vi "BRig_RT__Case_Idle__calc_LaserPulse.vi"(4 "input_dataExp_L_Tshutter":i32, 6 "input_dataExp_L_Tpeak":i32, 8 "input_dataExp_L_T":i32, 9 "input_dataExp_L_freq":i32, 11 "input_dataExp":u16[](array[numeric])) -> (2 "output_cluster":cluster{u16[], u16[]})   [LabVIEW 2014]
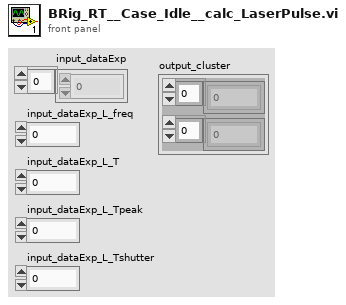
[diagram p1: front panel]
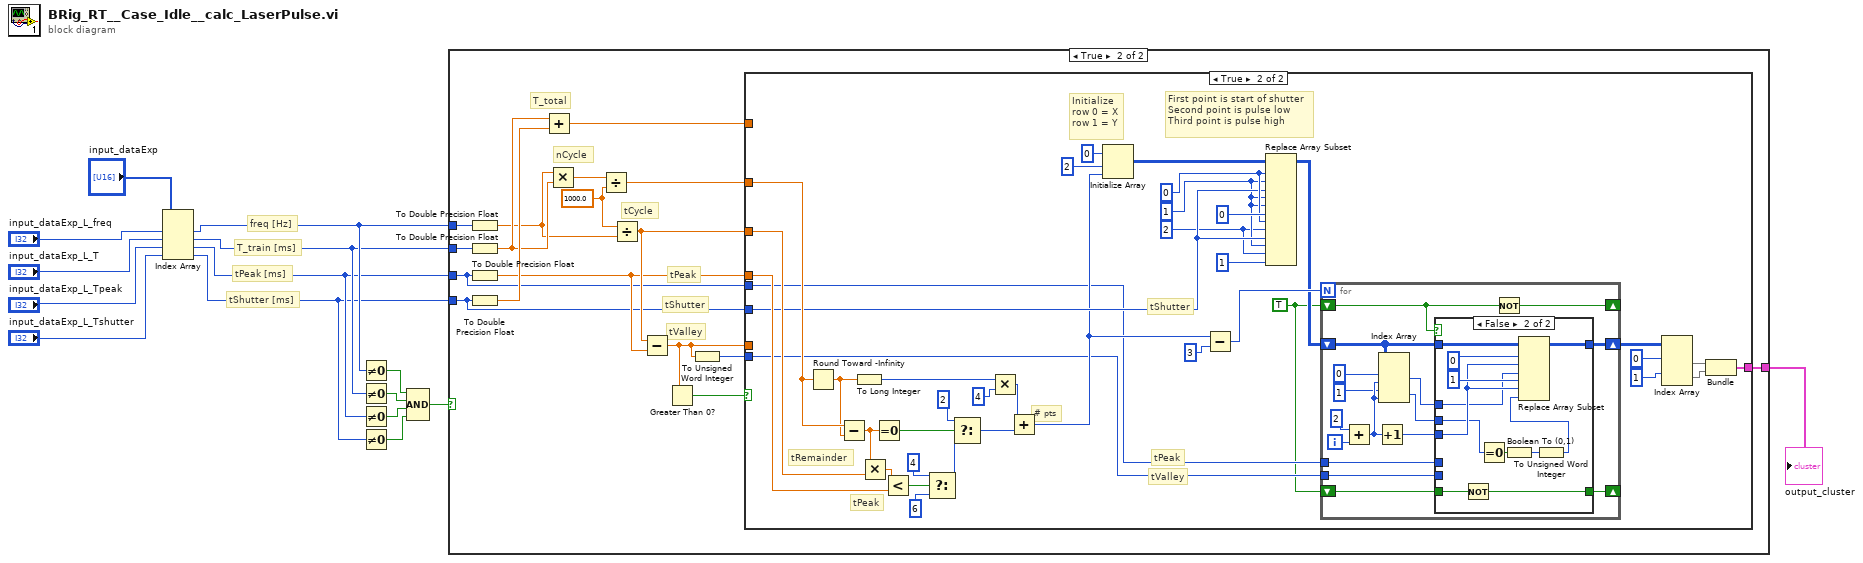
[diagram p0: block diagram]
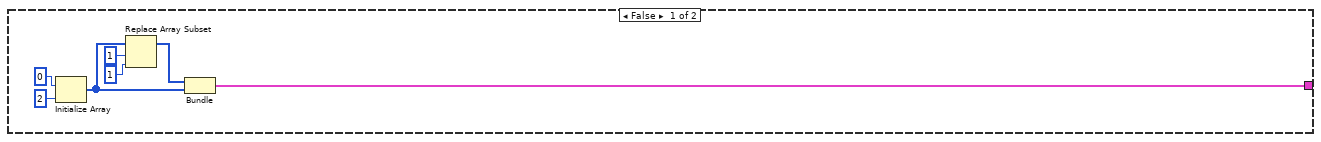
[diagram p2: hidden frame]
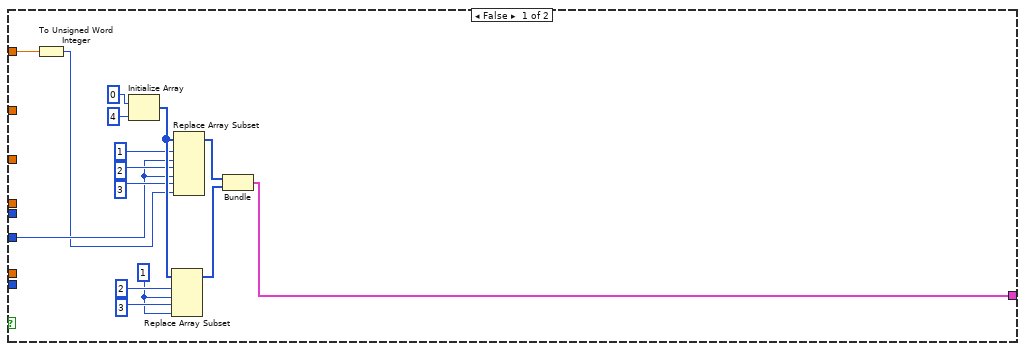
[diagram p3: hidden frame]
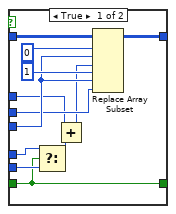
[diagram p4: hidden frame]
diagram:
  # "tShutter [ms]"
  # "tPeak [ms]"
  # "T_train [ms]"
  # "freq [Hz]"
  n1 = Index Array(array="input_dataExp", index #1="input_dataExp_L_freq", index #2="input_dataExp_L_T", index #3="input_dataExp_L_Tpeak", index #4="input_dataExp_L_Tshutter") -> (element #1=w8:u16, element #2=w7:u16, element #3=w6:u16, element #4=w5:u16)
  n2 = Not Equal To 0?(x=w8) -> (x != 0?=w14:bool)
  n3 = Not Equal To 0?(x=w7) -> (x != 0?=w13:bool)
  n4 = Not Equal To 0?(x=w6) -> (x != 0?=w12:bool)
  n5 = Not Equal To 0?(x=w5) -> (x != 0?=w11:bool)
  n6 = Compound Arithmetic op=AND(w14, w13, w12, w11) -> (w10:bool)
  n7 = case shown="True" w10 {
    tunnel: w8 -> [_ w34]
    tunnel: w7 -> [_ w33]
    tunnel: w6 -> [_ w26]
    tunnel: w5 -> [_ w27]
    tunnel: [w16 w23] -> w9
    frame False {
      n8 = Initialize Array(u16 0 ("element"), 2 ("dimension size")) -> (w20:u16[])
      n9 = Replace Array Subset(array=w20, new element=u16 1 ("new element/subarray"), index=1) -> (w17:u16[])
      n10 = Bundle(w17, w20) -> (w16:cluster{u16[], u16[]})  [unwired: 1 in]
    }
    frame True {
      w36 = 1000.0 ("y")
      # "tShutter"
      # "tPeak"
      # "tValley"
      # "tCycle"
      # "nCycle"
      # "T_total"
      n11 = To Double Precision Float(number=w34) -> (double precision float=w35:dbl)
      n12 = To Double Precision Float(number=w33) -> (double precision float=w38:dbl)
      n13 = To Double Precision Float(number=w26) -> (double precision float=w28:dbl)
      n14 = To Double Precision Float(number=w27) -> (double precision float=w39:dbl)
      n15 = Add(x=w38, y=w39) -> (x+y=w29:dbl)
      n16 = Multiply(x=w35, y=w38) -> (x*y=w37:dbl)
      n17 = Divide(x=w37, y=w36) -> (x/y=w30:dbl)
      n18 = Divide(x=w36, y=w35) -> (x/y=w31:dbl)
      n19 = Subtract(x=w31, y=w28) -> (x-y=w25:dbl)
      n20 = Greater Than 0?(x=w25) -> (x > 0?=w32:bool)
      n21 = To Unsigned Word Integer(number=w25) -> (unsigned 16bit integer=w24:u16)
      n22 = case shown="True" w32 {
        tunnel: w25 -> [_ _]
        tunnel: w31 -> [_ w89]
        tunnel: w30 -> [_ w79]
        tunnel: w29 -> [w43 _]
        tunnel: w28 -> [_ w87]
        tunnel: w27 -> [w44 w71]
        tunnel: w26 -> [_ w63]
        tunnel: w24 -> [_ w62]
        tunnel: [w40 w55] -> w23
        frame False {
          w50 = u16 1 ("new element/subarray")
          n23 = To Unsigned Word Integer(number=w43) -> (unsigned 16bit integer=w42:u16)
          n24 = Initialize Array(u16 0 ("element"), 4 ("dimension size")) -> (w48:u16[])
          n25 = Replace Array Subset(array=w48, new element #1=w50, index #1=2 ("index"), new element #2=w50, index #2=3 ("index")) -> (w49:u16[])
          n26 = Replace Array Subset(array=w48, new element #1=w44, index #1=1 ("new element/subarray"), new element #2=w44, index #2=2 ("index"), new element #3=w42, index #3=3 ("index")) -> (w41:u16[])
          n27 = Bundle(w41, w49) -> (w40:cluster{u16[], u16[]})  [unwired: 1 in]
        }
        frame True {
          w61 = TRUE
          w69 = 2 ("disabled index (col)")
          w70 = 1 ("dimension size")
          w72 = 0 ("dimension size")
          # "tValley"
          # "tPeak"
          # "tShutter"
          # "First point is start of shutter\nSecond point is pulse low\nThird point is pulse high"
          # "Initialize\nrow 0 = X\nrow 1 = Y"
          # "tPeak"
          # "tRemainder"
          # "# pts"
          n28 = Round Toward -Infinity(1:w79) -> (0:w78:dbl)
          n29 = Subtract(x=w79, y=w78) -> (x-y=w90:dbl)
          n30 = To Long Integer(number=w78) -> (32bit integer=w77:i32)
          n31 = Multiply(x=w90, y=w89) -> (x*y=w88:dbl)
          n32 = Equal To 0?(x=w90) -> (x = 0?=w92:bool)
          n33 = Less?(x=w88, y=w87) -> (x < y?=w86:bool)
          n34 = Select(t=4, s=w86, f=6) -> (s? t:f=w83:i32)
          n35 = Select(t=2, s=w92, f=w83) -> (s? t:f=w81:i32)
          n36 = Multiply(x=w77, y=4) -> (x*y=w80:i32)
          n37 = Add(x=w80, y=w81) -> (x+y=w67:i32)
          n38 = Initialize Array(u16 0 ("element"), 2 ("dimension size"), w67) -> (w74:u16[][])
          n39 = Subtract(x=w67, y=3) -> (x-y=w66:i32)
          n40 = Replace Array Subset(array=w74, new element #1=w71, index (row) #1=w72, index (col) #1=w70, new element #2=u16 0 ("new element/subarray"), index (row) #2=w70, index (col) #2=w70, new element #3=w71, index (row) #3=w72, index (col) #3=w69, new element #4=u16 1 ("new element/subarray"), index (row) #4=w70, index (col) #4=w69) -> (w64:u16[][])
          n41 = for {
            N: w66 -> [_]
            shift-right: [w93] -> w60
            shift-left: w64 -> [w101]
            tunnel: w63 -> [w97]
            tunnel: w62 -> [w96]
            shift-right: [w103] -> _
            shift-left: w61 -> [w102]
            shift-right: [w94] -> _
            shift-left: w61 -> [w95]
            i -> [w108]
            n42 = Add(x=2, y=w108) -> (x+y=w106:i32)
            n43 = Increment(x=w106) -> (x+1=w98:i32)
            n44 = Index Array(array=w101, index (row) #1=0 ("dimension size"), index (col) #1=w106, index (row) #2=1 ("dimension size"), index (col) #2=w106) -> (element #1=w100:u16, element #2=w99:u16)
            n45 = case shown="False" w102 {
              tunnel: w101 -> [w118 w130]
              tunnel: w100 -> [w113 w124]
              tunnel: w99 -> [w114 w123]
              tunnel: w98 -> [w115 w127]
              tunnel: w97 -> [w119 _]
              tunnel: w96 -> [w120 _]
              tunnel: w95 -> [w109 w131]
              tunnel: [w109 w132] -> w94
              tunnel: [w110 w126] -> w93
              frame True {
                n46 = Select(t=w119, s=w109, f=w120) -> (s? t:f=w112:u16)
                n47 = Add(x=w113, y=w112) -> (x+y=w111:u16)
                n48 = Replace Array Subset(array=w118, new element #1=w111, index (row) #1=0 ("dimension size"), index (col) #1=w115, new element #2=w114, index (row) #2=1 ("dimension size"), index (col) #2=w115) -> (w110:u16[][])
              }
              frame False {
                n49 = Not(x=w131) -> (.not. x?=w132:bool)
                n50 = Equal To 0?(x=w123) -> (x = 0?=w125:bool)
                n51 = Boolean To (0,1)(Boolean=w125) -> (0, 1=w122:i16)
                n52 = To Unsigned Word Integer(number=w122) -> (unsigned 16bit integer=w121:u16)
                n53 = Replace Array Subset(array=w130, new element #1=w124, index (row) #1=0 ("dimension size"), index (col) #1=w127, new element #2=w121, index (row) #2=1 ("dimension size"), index (col) #2=w127) -> (w126:u16[][])
              }
            }
            n54 = Not(x=w102) -> (.not. x?=w103:bool)
          }
          n55 = Index Array(array=w60, index (row) #1=0 ("dimension size"), index (row) #2=1 ("dimension size")) -> (element #1=w57:u16[], element #2=w56:u16[])  [unwired: 2 in]
          n56 = Bundle(w57, w56) -> (w55:cluster{u16[], u16[]})  [unwired: 1 in]
        }
      }
    }
  }
  "output_cluster" <- w9
